vi "register.events.vi"(8 "error in (no error)":errorcluster, 11 "EventDaemon in":refnum<class "ErrorHandler.lvclass">) -> (0 "error out":errorcluster, 2 "Event Registration Refnum":refnum<event-registration>, 3 "EventDaemon out":refnum<class "ErrorHandler.lvclass">)   [LabVIEW 2024, in "ErrorHandler.lvclass"]
doc: "Registers all events in the event--cluster.ctl"
uses:
  ErrorHandler.lvclass
  ErrorHandler.lvclass/ErrorHandler.ctl
  events--cluster.ctl
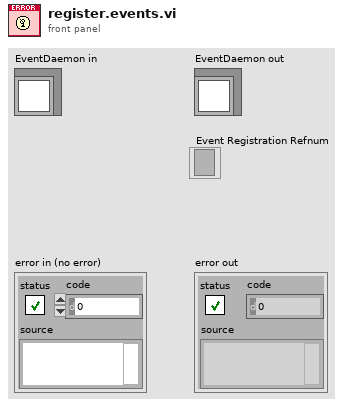
[diagram p1: front panel]
types:
  T1 = typedef "ErrorHandler.lvclass/events--cluster.ctl" = cluster{"exit event":refnum<user-event>, "period event":refnum<user-event>, "error event":refnum<user-event>}
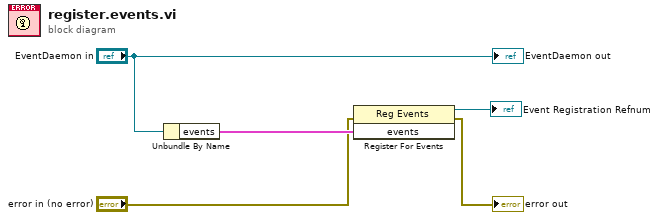
[diagram p0: block diagram]
diagram:
  n1 = Unbundle By Name("EventDaemon in") -> ("events"=w5:T1)
  n2 = register-events(error in="error in (no error)", w5) -> (reference out=→"Event Registration Refnum":refnum<event-registration>, error out=→"error out":errorcluster)  [unwired: 1 in]
  "EventDaemon out" <- "EventDaemon in"
